vi "Initialize Address_Index Lists.vi"(8 "error in":errorcluster, 10 "group name":string, 11 "tag list":T4[](array[typedef])) -> (0 "error out":errorcluster, 3 "config server message":T1)   [LabVIEW 2010, in "NI_CCC.lvlib"]
uses:
  NI_CCC.lvlib
  Tag Configuration.ctl
  <vilib>/NI/Current Value Table/Type Defs/Data Types.ctl
  Tag Direction.ctl
  Configure Read_Write Message.ctl
  Type_Tag.ctl
  <vilib>/NI/Current Value Table/FGVs/Group Memory Methods.ctl
  <vilib>/NI/Current Value Table/FGVs/Tag Memory.vi
  <vilib>/NI/Current Value Table/Form Single Group.vi
  <vilib>/NI/Current Value Table/Current Value Table.lvlib
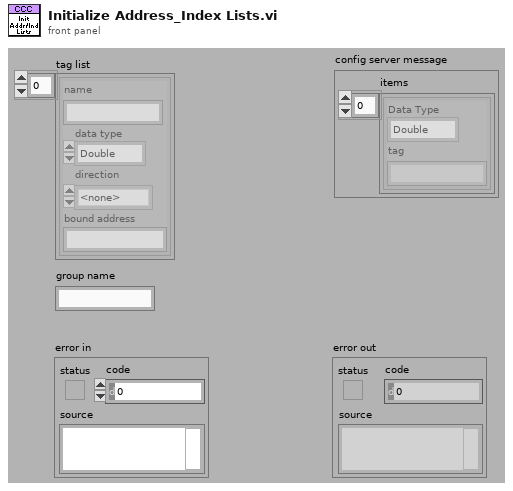
[diagram p1: front panel]
types:
  T1 = typedef "NI_CCC.lvlib/Configure Read_Write Message.ctl" = cluster{"items":T2[]}
  T2 = typedef "NI_CCC.lvlib/Type_Tag.ctl" = cluster{"Data Type":T3, "tag":string}
  T3 = typedef "Current Value Table.lvlib/Data Types.ctl" = enum16{"Double", "Single", "I64", "I32", "I16", "I8", "U64", "U32", "U16", "U8", "String", "Boolean", "Array of U8", "Array of U16", "Array of U32", "Array of U64", "Array of I64", "Array of I32", "Array of I16", "Array of I8", "Array of Double", "Array of Single", "Array of Boolean", "Array of String"}
  T4 = typedef "NI_CCC.lvlib/Tag Configuration.ctl" = cluster{"name":string, "data type":T3, "direction":T5, "bound address":string}
  T5 = typedef "NI_CCC.lvlib/Tag Direction.ctl" = enum32{"<none>", "Read", "Write"}
  T6 = typedef "Current Value Table.lvlib/Group Memory Methods.ctl" = enum16{"Clear", "Read Indices in Group", "List Groups", "List Tags by Type", "List Tags", "Delete Group", "Check Group Existence", "Create Group"}
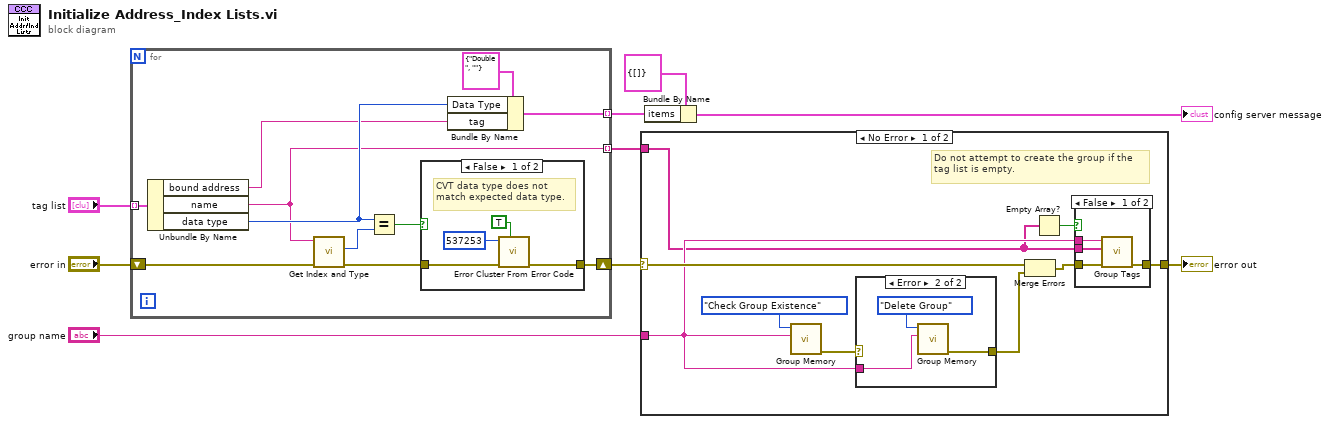
[diagram p0: block diagram]
diagram:
  n1 = for {
    tunnel: "tag list" -> [w20] mode=indexing
    shift-right: [w15] -> w3
    shift-left: "error in" -> [w19]
    tunnel: [w11] -> w6 mode=indexing
    tunnel: [w10] -> w1 mode=indexing
    n2 = Unbundle By Name(w20) -> ("bound address"=w12:string, "name"=w10:string, "data type"=w13:T3)
    n3 = call <vilib>:"Get Index and Type.vi"("error in (no error)"=w19, "Tag"=w10) -> ("error out"=w16:errorcluster, "Type"=w18:T3)  [unwired: 7 in, 1 out]
    n4 = Equal?(x=w13, y=w18) -> (x = y?=w17:bool)
    n5 = case shown="False" w17 {
      tunnel: w16 -> [w23 w25]
      tunnel: [w22 w25] -> w15
      frame False {
        # "CVT data type does not match expected data type."
        n6 = call <vilib>:"Error Cluster From Error Code.vi"("show call chain? (False)"=TRUE, "error in (no error)"=w23, "error code (0)"=537253) -> ("error out"=w22:errorcluster)  [unwired: 6 out]
      }
      frame True {
      }
    }
    n7 = Bundle By Name(cluster=T2 {"Data Type"=enum."Double", "tag"=""} ("type_tag"), "Data Type"=w13, "tag"=w12) -> (w11:T2)
  }
  n8 = case shown="No Error" w3 {
    selector: w3 -> [w30 w44]
    tunnel: "group name" -> [w29 _]
    tunnel: [w28 w44] -> w2
    tunnel: w1 -> [w27 _]
    frame No Error {
      # "Do not attempt to create the group if the tag list is empty."
      n9 = call <vilib>:"Group Memory.vi"("Group"=w29, "Method"=Group_Memory_Methods."Check Group Existence") -> ("error out"=w32:errorcluster)  [unwired: 6 in, 3 out]
      n10 = case shown="Error" w32 {
        selector: w32 -> [w40 _]
        tunnel: w29 -> [_ w42]
        tunnel: [w40 w41] -> w33
        frame No Error {
        }
        frame Error {
          n11 = call <vilib>:"Group Memory.vi"("Group"=w42, "Method"=Group_Memory_Methods."Delete Group") -> ("error out"=w41:errorcluster)  [unwired: 6 in, 3 out]
        }
      }
      n12 = Merge Errors(w30, w33) -> (w34:errorcluster)
      n13 = Empty Array?(array=w27) -> (empty?=w26:bool)
      n14 = case shown="False" w26 {
        tunnel: w34 -> [w38 w39]
        tunnel: w29 -> [w37 _]
        tunnel: [w36 w39] -> w28
        tunnel: w27 -> [w35 _]
        frame False {
          n15 = call <vilib>:"Group Tags.vi"("error in (no error)"=w38, "Tag Names"=w35, "Group"=w37) -> ("error out"=w36:errorcluster)  [unwired: 8 in]
        }
        frame True {
        }
      }
    }
    frame Error {
    }
  }
  "error out" <- w2
  n16 = Bundle By Name(cluster=T1 {"items"=[]} ("config write message"), "items"=w6) -> (→"config server message":T1)
